vi "PUEBAARRAYfOR.vi"() -> ()   [LabVIEW 2018]
uses:
  <vilib>/Utility/file.llb/Read Delimited Spreadsheet (DBL).vi
panel:
  out "element 2":dbl
  in  "tiempo":dbl
  out "element":dbl
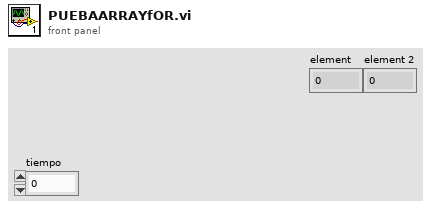
[diagram p1: front panel]
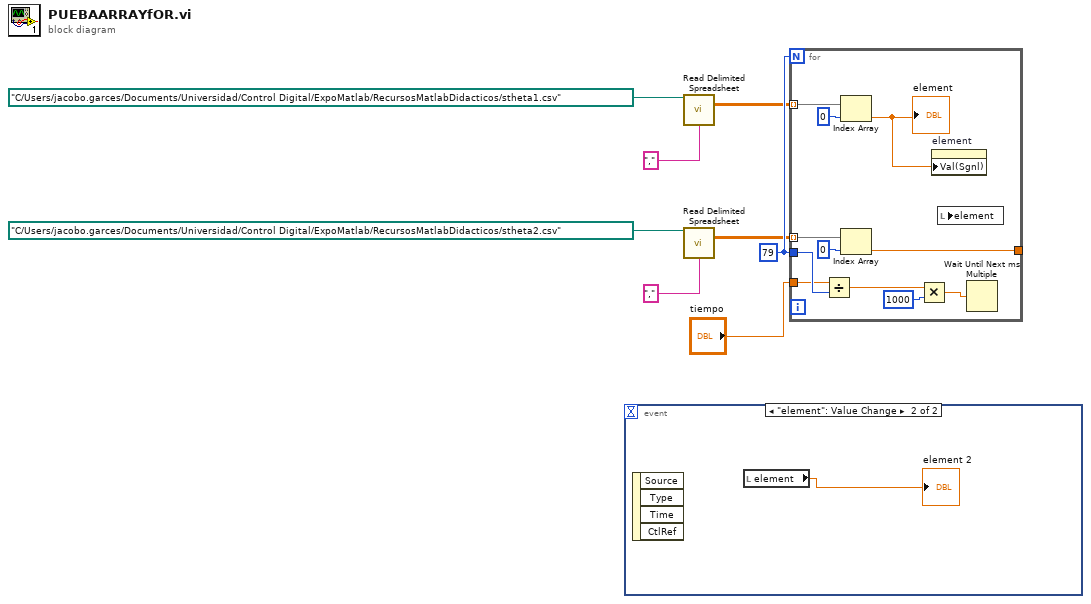
[diagram p0: block diagram]
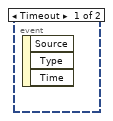
[diagram p2: hidden frame]
diagram:
  w6 = 79
  n1 = event shown="[1] \"element\": Value Change" {
    selector: _ -> [_ _]
    dyn-events: _ -> [_ _]
    timeout: _ -> [_ _]
    event Timeout {
      n2 = event-data() -> ()  [unwired: 1 in, 3 out]
    }
    event "element": Value Change {
      n3 = event-data() -> ()  [unwired: 1 in, 4 out]
      n4 = local read "element"() -> (→"element 2":dbl)
    }
  }
  n5 = call-poly <vilib>:"Read Delimited Spreadsheet.vi"("file path (dialog if empty)"=path "C:/Users/jacobo.garces/Documents/Universidad/Control Digital/ExpoMatlab/RecursosMatlabDidacticos/stheta1.csv", "delimiter (\\t)"="," ("delimiter (\\t)")) -> ("all rows"=w5:dbl[][])  [unwired: 8 in, 5 out]
  n6 = call-poly <vilib>:"Read Delimited Spreadsheet.vi"("file path (dialog if empty)"=path "C:/Users/jacobo.garces/Documents/Universidad/Control Digital/ExpoMatlab/RecursosMatlabDidacticos/stheta2.csv", "delimiter (\\t)"="," ("delimiter (\\t)")) -> ("all rows"=w3:dbl[][])  [unwired: 8 in, 5 out]
  n7 = for {
    N: w6 -> [_]
    tunnel: w6 -> [w18]
    tunnel: w5 -> [w17] mode=indexing
    tunnel: "tiempo" -> [w15]
    tunnel: w3 -> [w13] mode=indexing
    tunnel: [w12] -> _
    n8 = Divide(x=w15, y=w18) -> (x/y=w20:dbl)
    n9 = Index Array(array=w17, index=0) -> (element=w10:dbl)
    "element" <- w10
    n10 = Index Array(array=w13, index=0) -> (element=w12:dbl)
    n11 = Multiply(x=w20, y=1000) -> (x*y=w11:dbl)
    n12 = property on="element" class="DigNum (strict)"("Val(Sgnl)"=w10) -> ()  [unwired: 2 in, 2 out]
    n13 = local read "element"() -> ()  [unwired: 1 in]
    n14 = Wait Until Next ms Multiple(millisecond multiple=w11) -> ()  [unwired: 1 out]
  }
